vi "数据处理组合.vi"(11 "待排序数组":string[][][](array[string])) -> (3 "输出簇":T1)   [LabVIEW 2016]
uses:
  <userlib>/_OpenG.lib/array/array.llb/Remove Duplicates from 1D Array (String)__ogtk.vi
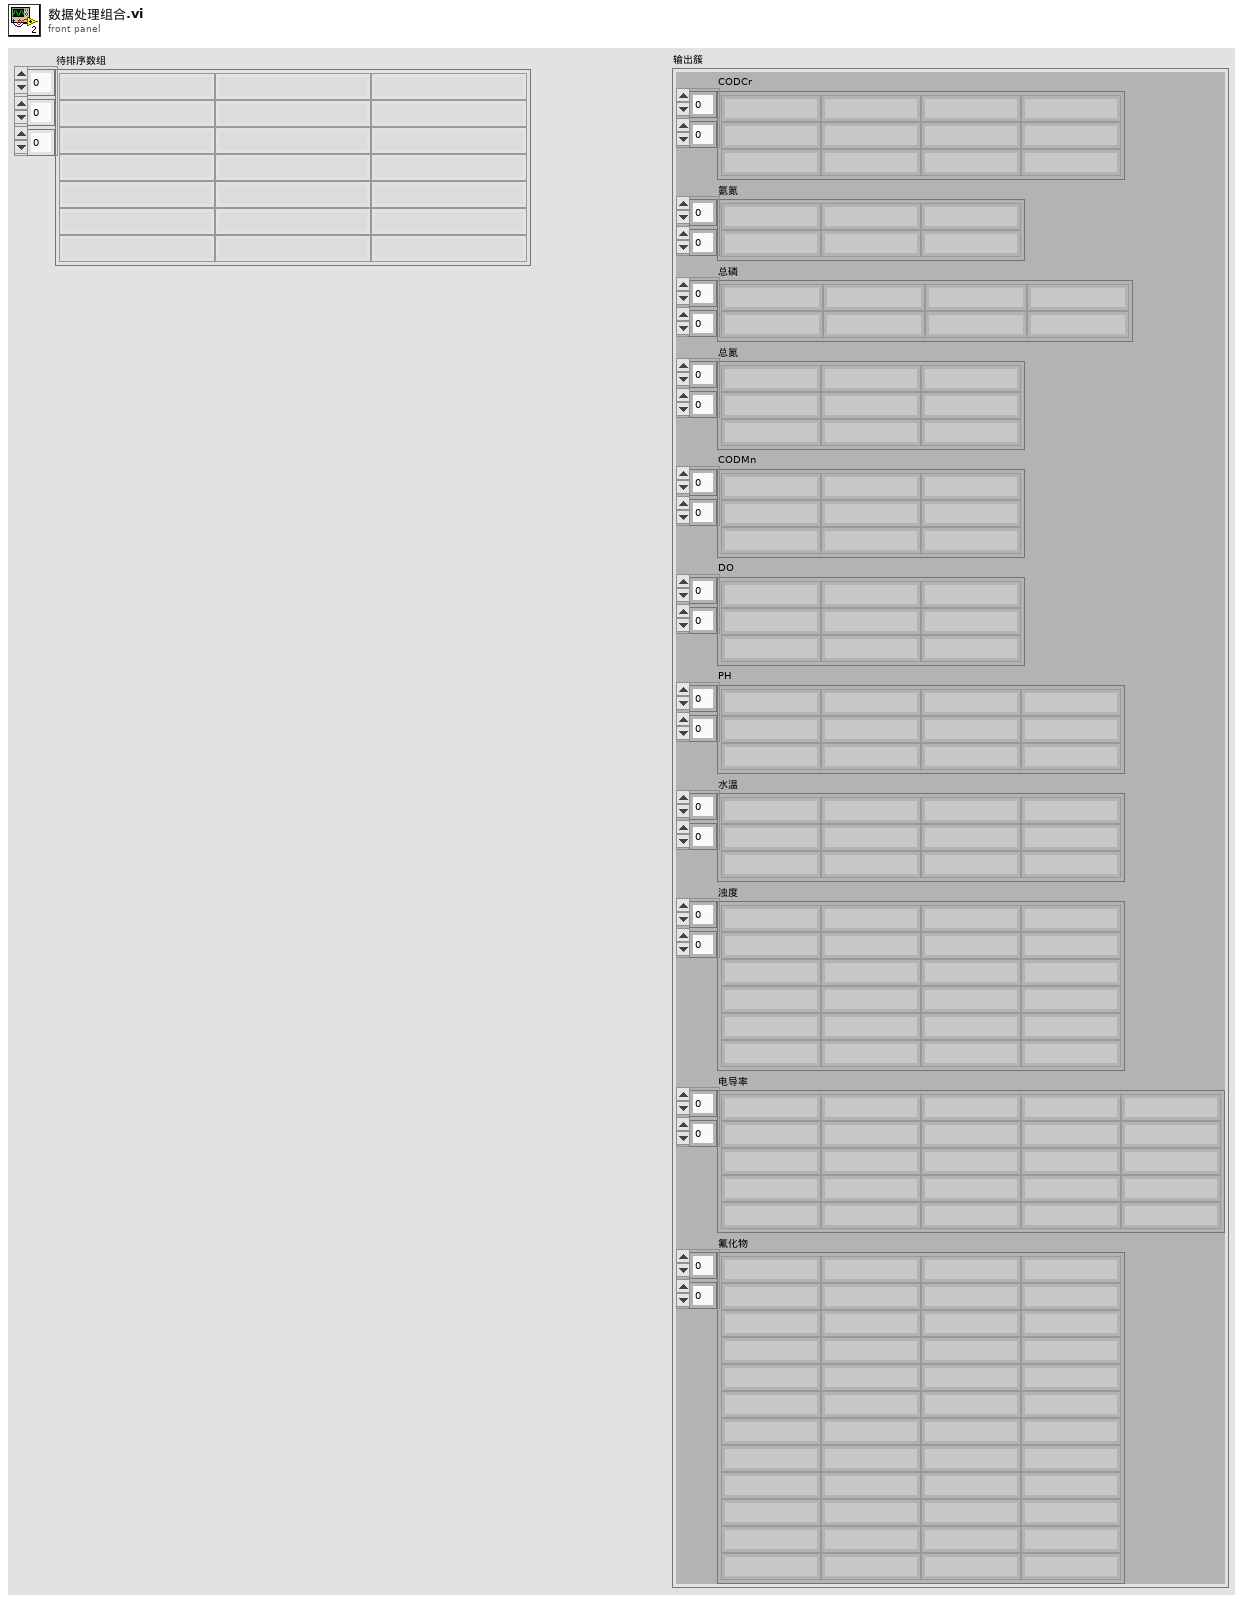
[diagram p1: front panel]
types:
  T1 = cluster{"CODCr":string[][], "氨氮":string[][], "总磷":string[][], "总氮":string[][], "CODMn":string[][], "DO":string[][], "PH":string[][], "水温":string[][], "浊度":string[][], "电导率":string[][], "氟化物":string[][]}
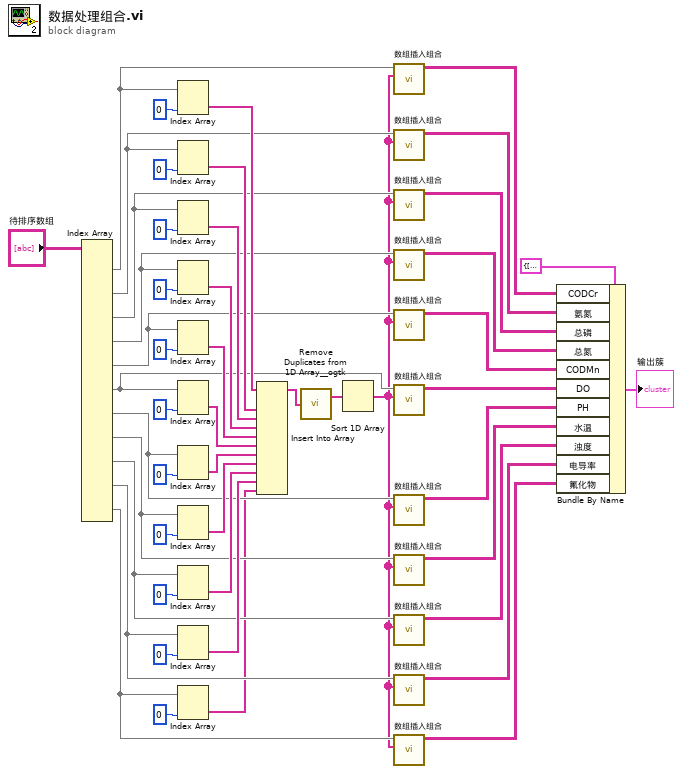
[diagram p0: block diagram]
diagram:
  n1 = Index Array(array="待排序数组") -> (element #1=w25:string[][], element #2=w24:string[][], element #3=w22:string[][], element #4=w20:string[][], element #5=w17:string[][], element #6=w15:string[][], element #7=w13:string[][], element #8=w11:string[][], element #9=w10:string[][], element #10=w9:string[][], element #11=w3:string[][])  [unwired: 33 in]
  n2 = Index Array(array=w25, index (col)=0 ("索引 (行)")) -> (element=w49:string[])  [unwired: 1 in]
  n3 = Index Array(array=w24, index (col)=0 ("索引 (行)")) -> (element=w47:string[])  [unwired: 1 in]
  n4 = Index Array(array=w22, index (col)=0 ("索引 (行)")) -> (element=w43:string[])  [unwired: 1 in]
  n5 = Index Array(array=w20, index (col)=0 ("索引 (行)")) -> (element=w42:string[])  [unwired: 1 in]
  n6 = Index Array(array=w17, index (col)=0 ("索引 (行)")) -> (element=w41:string[])  [unwired: 1 in]
  n7 = Index Array(array=w15, index (col)=0 ("索引 (行)")) -> (element=w39:string[])  [unwired: 1 in]
  n8 = Index Array(array=w13, index (col)=0 ("索引 (行)")) -> (element=w37:string[])  [unwired: 1 in]
  n9 = Index Array(array=w11, index (col)=0 ("索引 (行)")) -> (element=w35:string[])  [unwired: 1 in]
  n10 = Index Array(array=w10, index (col)=0 ("索引 (行)")) -> (element=w33:string[])  [unwired: 1 in]
  n11 = Index Array(array=w9, index (col)=0 ("索引 (行)")) -> (element=w31:string[])  [unwired: 1 in]
  n12 = Index Array(array=w3, index (col)=0 ("索引 (行)")) -> (element=w4:string[])  [unwired: 1 in]
  n13 = Insert Into Array(array=w49, new element #1=w47, new element #2=w43, new element #3=w42, new element #4=w41, new element #5=w39, new element #6=w37, new element #7=w35, new element #8=w33, new element #9=w31, new element #10=w4) -> (w26:string[])  [unwired: 1 in]
  n14 = call-poly <userlib>:"Remove Duplicates from 1D Array__ogtk.vi"("Input Array"=w26) -> ("Output Array"=w29:string[])  [unwired: 1 out]
  n15 = Sort 1D Array(array=w29) -> (sorted array=w2:string[])
  n16 = call "数组插入组合.vi"("排序后的一维数组"=w2, "输入数组"=w25) -> ("输出结果"=w27:string[][])  [unwired: 9 in]
  n17 = call "数组插入组合.vi"("排序后的一维数组"=w2, "输入数组"=w24) -> ("输出结果"=w23:string[][])  [unwired: 9 in]
  n18 = call "数组插入组合.vi"("排序后的一维数组"=w2, "输入数组"=w22) -> ("输出结果"=w21:string[][])  [unwired: 9 in]
  n19 = call "数组插入组合.vi"("排序后的一维数组"=w2, "输入数组"=w20) -> ("输出结果"=w19:string[][])  [unwired: 9 in]
  n20 = call "数组插入组合.vi"("排序后的一维数组"=w2, "输入数组"=w17) -> ("输出结果"=w16:string[][])  [unwired: 9 in]
  n21 = call "数组插入组合.vi"("排序后的一维数组"=w2, "输入数组"=w15) -> ("输出结果"=w14:string[][])  [unwired: 9 in]
  n22 = call "数组插入组合.vi"("排序后的一维数组"=w2, "输入数组"=w13) -> ("输出结果"=w12:string[][])  [unwired: 9 in]
  n23 = call "数组插入组合.vi"("排序后的一维数组"=w2, "输入数组"=w11) -> ("输出结果"=w8:string[][])  [unwired: 9 in]
  n24 = call "数组插入组合.vi"("排序后的一维数组"=w2, "输入数组"=w10) -> ("输出结果"=w7:string[][])  [unwired: 9 in]
  n25 = call "数组插入组合.vi"("排序后的一维数组"=w2, "输入数组"=w9) -> ("输出结果"=w6:string[][])  [unwired: 9 in]
  n26 = call "数组插入组合.vi"("排序后的一维数组"=w2, "输入数组"=w3) -> ("输出结果"=w1:string[][])  [unwired: 9 in]
  n27 = Bundle By Name(cluster=T1 {"CODCr"=[], "氨氮"=[], "总磷"=[], "总氮"=[], "CODMn"=[], "DO"=[], "PH"=[], "水温"=[], "浊度"=[], "电导率"=[], "氟化物"=[]}, "CODCr"=w27, "氨氮"=w23, "总磷"=w21, "总氮"=w19, "CODMn"=w16, "DO"=w14, "PH"=w12, "水温"=w8, "浊度"=w7, "电导率"=w6, "氟化物"=w1) -> (→"输出簇":T1)
